vi "Video stream.vi"(4 "Write video":bool, 6 "Video name":string="test", 7 "Interface name":T1="cam0", 8 "Video directory path":path=path "C:/test", 9 "FPS":u32=30, 10 "Video codec":string="Microsoft Video 1", 11 "VideoMode":u32) -> (0 "Error Out":errorcluster)   [LabVIEW 2014]
uses:
  <vilib>/userdefined/High Color/IMAQdx.ctl
  <vilib>/vision/driver/IMAQdx.llb/IMAQdx Camera Control Mode.ctl
  <vilib>/vision/Avi.llb/IMAQ AVI2 Refnum.ctl
  <vilib>/vision/driver/NI_Vision_Acquisition_Software.lvlib
  <resource>/objmgr/imaqdx.rc
panel:
  in  "Stop":bool
  out "Image":T2(plugin-control)
  # "PN 27/11/2014"
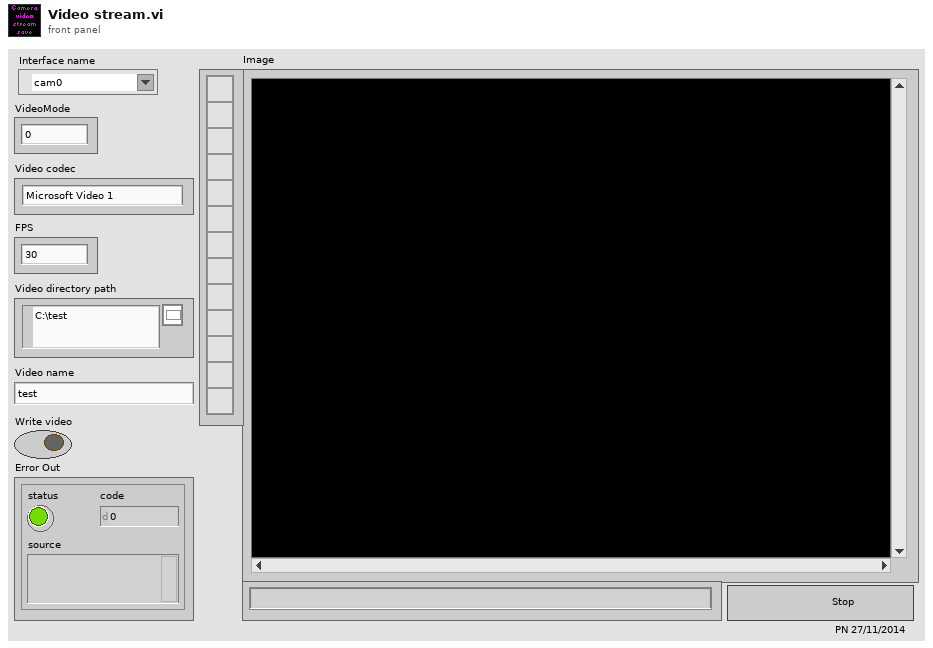
[diagram p1: front panel]
types:
  T1 = typedef "IMAQdx.ctl" = refnum<k21>
  T2 = typedef "IMAQ Image.ctl" = refnum<image>
  T3 = typedef "NI_Vision_Acquisition_Software.lvlib/IMAQdx Camera Control Mode.ctl" = enum32{"Controller", "Listener"}
  T4 = typedef "IMAQ AVI2 Refnum.ctl" = refnum<k20>
  T5 = typedef "Image Type" = u32
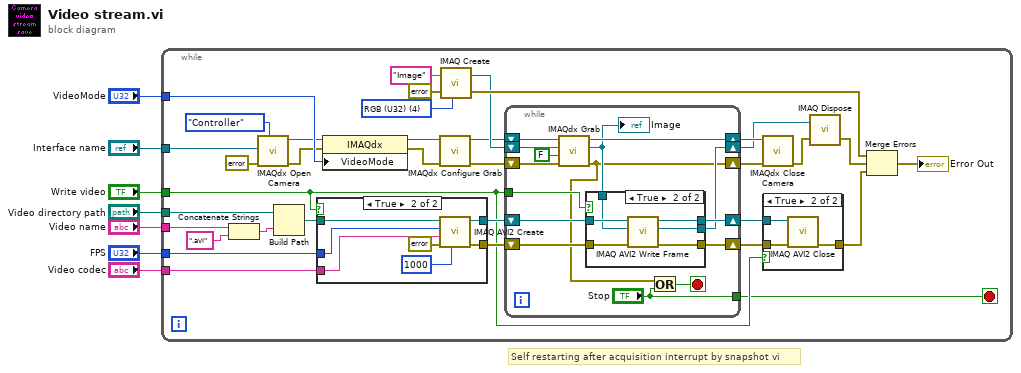
[diagram p0: block diagram]
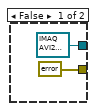
[diagram p2: hidden frame]
diagram:
  # "Self restarting after acquisition interrupt by snapshot vi"
  n1 = while {
    tunnel: "Video directory path" -> [w41]
    tunnel: "Video name" -> [w39]
    tunnel: "Write video" -> [w20]
    tunnel: "VideoMode" -> [w19]
    tunnel: "FPS" -> [w14]
    tunnel: "Interface name" -> [w13]
    tunnel: "Video codec" -> [w11]
    stop <- w10 stop-if-true
    w36 = T5 4 items=["Grayscale (U8)", "Grayscale (I16)", "Grayscale (SGL)", "Complex (CSG)", "RGB (U32)", "HSL (U32)", "RGB (U64)", "Grayscale (U16)"] ("Image Type")
    n2 = Concatenate Strings(w39, ".avi" ("name or relative path")) -> (w38:string)
    n3 = call <vilib>:"IMAQdx Open Camera.vi"("Camera Control Mode"=IMAQdx_Camera_Control_Mode."Controller", "error in"=errorcluster {"status"=FALSE, "code"=0, "source"=""}, "Session In"=w13) -> ("error out"=w16:errorcluster, "Session Out"=w12:T1)  [unwired: 7 in]
    n4 = Build Path(base path=w41, name or relative path=w38) -> (appended path=w30:path)
    n5 = case shown="True" w20 {
      tunnel: w30 -> [_ w51]
      tunnel: [T4 refnum ("AVI Refnum") w49] -> w29
      tunnel: [errorcluster {"status"=FALSE, "code"=0, "source"=""} ("error out") w48] -> w28
      tunnel: w14 -> [_ w47]
      tunnel: w11 -> [_ w46]
      frame False {
      }
      frame True {
        n6 = call "IMAQ AVI2 Create"("Quality"=1000, "error in (no error)"=errorcluster {"status"=FALSE, "code"=0, "source"=""} ("error in"), "Codec"=w46, "Frames Per Second"=w47, "AVI Path"=w51) -> ("error out"=w48:errorcluster, "AVI Refnum"=w49:T4)  [unwired: 5 in]
      }
    }
    n7 = property class="IMAQdx"(reference=w12, error in=w16, "VideoMode"=w19) -> (reference out=w17:T1, error out=w15:errorcluster)
    n8 = call <vilib>:"IMAQdx Configure Grab.vi"("error in"=w15, "Session In"=w17) -> ("error out"=w31:errorcluster, "Session Out"=w18:T1)  [unwired: 8 in]
    n9 = call "IMAQ Create"("Image Name"="Image", "Image Type"=w36, "error in (no error)"=errorcluster {"status"=FALSE, "code"=0, "source"=""} ("error in")) -> ("New Image"=w34:T2, "error out"=w35:errorcluster)  [unwired: 2 in]
    n10 = while {
      shift-right: [w68] -> w33
      shift-left: w18 -> [w70]
      shift-right: [w60] -> w26
      shift-left: w34 -> [w69]
      shift-right: [w58] -> w32
      shift-left: w31 -> [w67]
      tunnel: w20 -> [w65]
      shift-right: [w62] -> w21
      shift-left: w29 -> [w64]
      shift-right: [w59] -> w23
      shift-left: w28 -> [w61]
      tunnel: ["Stop"] -> w10
      stop <- w57 stop-if-true
      n11 = call <vilib>:"IMAQdx Grab.vi"("error in"=w67, "Wait for Next Buffer? (Yes)"=FALSE, "Image In"=w69, "Session In"=w70) -> ("error out"=w58:errorcluster, "Image Out"=w63:T2, "Session Out"=w68:T1)  [unwired: 4 in, 1 out]
      "Image" <- w63
      n12 = case shown="True" w65 {
        tunnel: w64 -> [w73 w79]
        tunnel: w63 -> [w71 w78]
        tunnel: [w73 w77] -> w62
        tunnel: [w72 w76] -> w59
        tunnel: w61 -> [w72 w75]
        tunnel: [w71 w74] -> w60
        frame False {
        }
        frame True {
          n13 = call "IMAQ AVI2 Write Frame"("error in (no error)"=w75, "Image"=w78, "AVI Refnum"=w79) -> ("error out"=w76:errorcluster, "Image Out (duplicate)"=w74:T2, "AVI Refnum (duplicate)"=w77:T4)  [unwired: 6 in]
        }
      }
      n14 = Or(x=w58, y="Stop") -> (x .or. y?=w57:bool)
    }
    n15 = call <vilib>:"IMAQdx Close Camera.vi"("error in"=w32, "Session In"=w33) -> ("error out"=w25:errorcluster)  [unwired: 9 in]
    n16 = case shown="True" w20 {
      tunnel: w23 -> [w52 w55]
      tunnel: [w52 w54] -> w22
      tunnel: w21 -> [_ w53]
      frame False {
      }
      frame True {
        n17 = call "IMAQ AVI2 Close"("error in (no error)"=w55, "AVI Refnum"=w53) -> ("error out"=w54:errorcluster)  [unwired: 9 in]
      }
    }
    n18 = call "IMAQ Dispose"("Image"=w26, "error in (no error)"=w25) -> ("error out"=w24:errorcluster)  [unwired: 4 in]
    n19 = Merge Errors(w35, w24, w22) -> (→"Error Out":errorcluster)
  }
